vi "AddRecordingOverlay2Image.vi"(8 "error in (no error)":errorcluster, 10 "Recording Status String":string, 11 "Input Image":T1) -> (0 "error out":errorcluster, 3 "Output Image":T1)   [LabVIEW 2013]
doc: "Use this template to build a VI to use as a subVI."
uses:
  <vilib>/vision/Image Controls.llb/IMAQ Image.ctl
panel:
  out "Reference Image":T1(plugin-control)
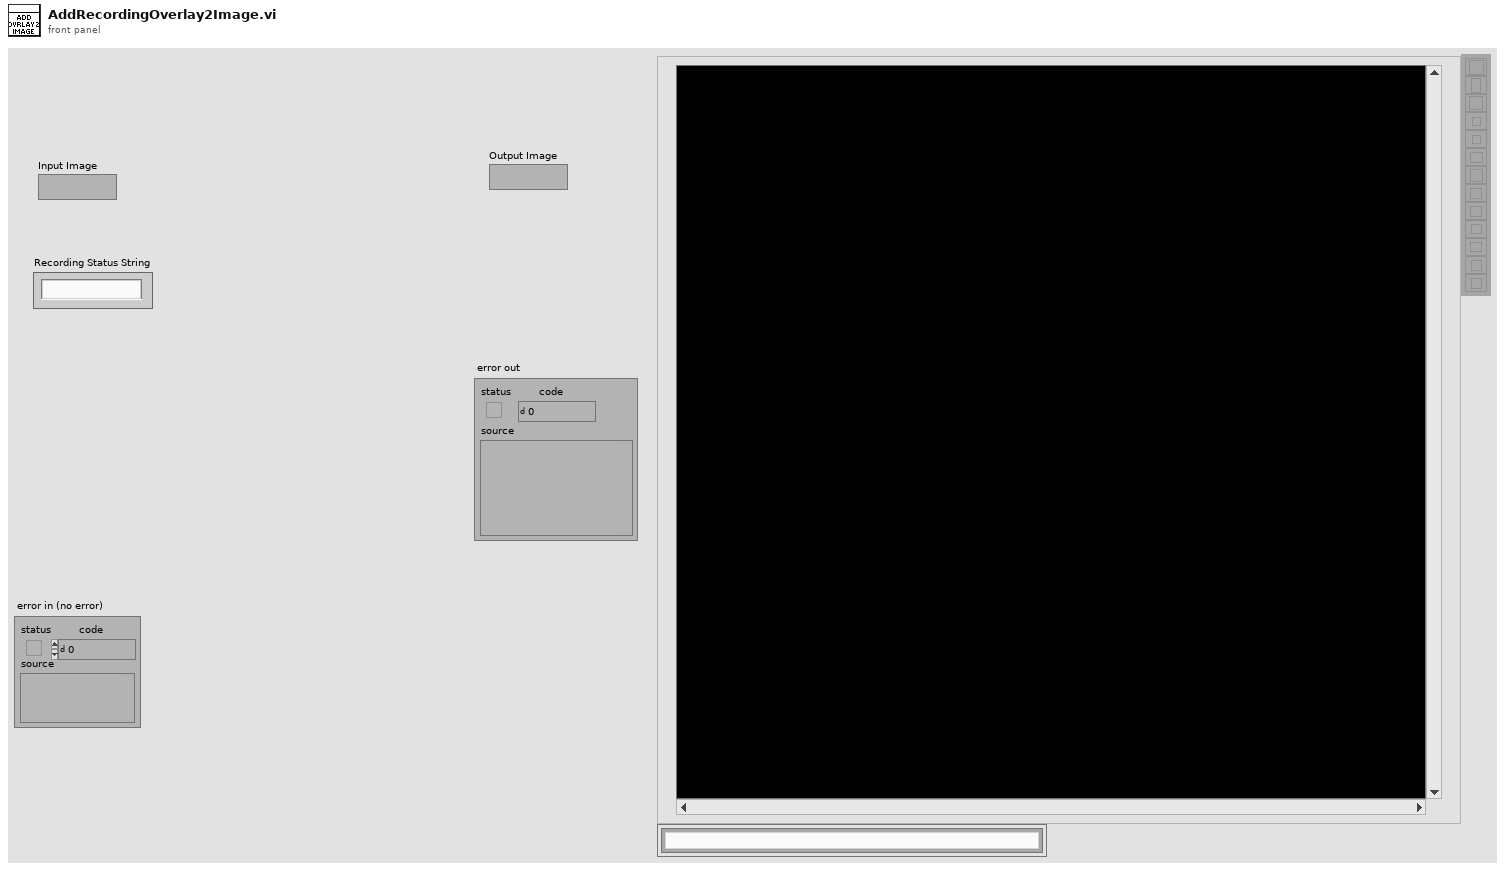
[diagram p1: front panel]
types:
  T1 = typedef "IMAQ Image.ctl" = refnum<image>
  T2 = cluster{"Left":i32, "Top":i32, "Right":i32, "Bottom":i32}
  T3 = cluster{"Desired Font (Application)":enum16{"User-specified Font", "Application Font", "System Font", "Dialog Font"}, "[User-specified Font]":cluster{"Font Name":string, "Size":i16, "Strikeout?":bool, "Italic?":bool, "Underline?":bool, "Outline?":bool, "Shadow?":bool, "Bold?":bool, "Rotation Angle":dbl}, "Horizontal Alignment":i16, "Vertical Alignment":i16}
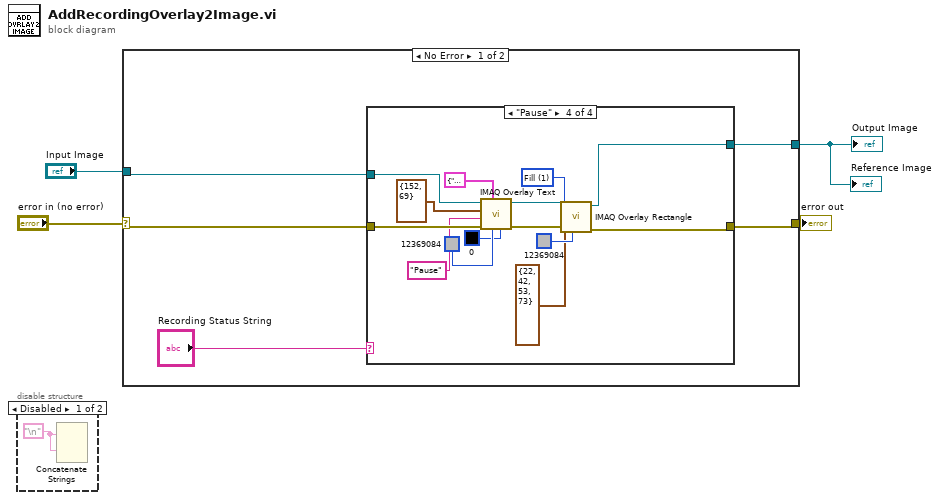
[diagram p0: block diagram]
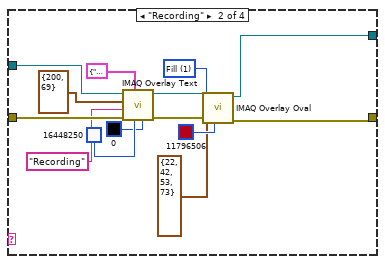
[diagram p4: hidden frame]
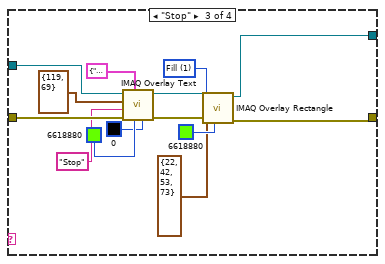
[diagram p5: hidden frame]
diagram:
  n1 = disable-structure shown="Disabled" {
    frame Disabled {
      w5 = "\n"
      n2 = Concatenate Strings(w5, w5) -> ()  [unwired: 3 in, 1 out]
    }
    frame Enabled {
    }
  }
  n3 = case shown="No Error" "error in (no error)" {
    selector: "error in (no error)" -> [w9 w55]
    tunnel: [w6 w55] -> w3
    tunnel: "Input Image" -> [w8 w54]
    tunnel: [w7 w54] -> w1
    frame No Error {
      n4 = case shown="\"Pause\"" "Recording Status String" {
        tunnel: w9 -> [_ w22 w36 w50]
        tunnel: w8 -> [w11 w21 w35 w49]
        tunnel: [w11 w15 w29 w43] -> w7
        tunnel: [_ w17 w31 w45] -> w6
        frame "False", Default {
        }
        frame "Recording" {
          w14 = u32 1 items=["Frame", "Fill"] ("Drawing Mode (Frame)")
          n5 = call "IMAQ Overlay Text"("BG Color (Transparent)"=u32 0, "Text Color (black)"=u32 16448250, "Font, Size & Style"=T3 {"Desired Font (Application)"=enum."User-specified Font", "[User-specified Font]"={"Font Name"="", "Size"=32, "Strikeout?"=FALSE, "Italic?"=FALSE, "Underline?"=FALSE, "Outline?"=FALSE, "Shadow?"=FALSE, "Bold?"=TRUE, "Rotation Angle"=0.0}, "Horizontal Alignment"=2, "Vertical Alignment"=2}, "error in (no error)"=w22, "String"="Recording", "Origin"=cluster{"X":i32, "Y":i32} {"X"=200, "Y"=69}, "Image"=w21) -> ("error out"=w18:errorcluster, "Image Out"=w16:T1)  [unwired: 3 in]
          n6 = call "IMAQ Overlay Oval"("Color"=u32 11796506, "error in (no error)"=w18, "Drawing Mode (Frame)"=w14, "Bounding Rectangle"=T2 {"Left"=22, "Top"=42, "Right"=53, "Bottom"=73}, "Image"=w16) -> ("error out"=w17:errorcluster, "Image Out"=w15:T1)  [unwired: 5 in]
        }
        frame "Stop" {
          w28 = u32 1 items=["Frame", "Fill"] ("Drawing Mode (Frame)")
          n7 = call "IMAQ Overlay Text"("BG Color (Transparent)"=u32 0, "Text Color (black)"=u32 6618880, "Font, Size & Style"=T3 {"Desired Font (Application)"=enum."User-specified Font", "[User-specified Font]"={"Font Name"="", "Size"=32, "Strikeout?"=FALSE, "Italic?"=FALSE, "Underline?"=FALSE, "Outline?"=FALSE, "Shadow?"=FALSE, "Bold?"=TRUE, "Rotation Angle"=0.0}, "Horizontal Alignment"=2, "Vertical Alignment"=2}, "error in (no error)"=w36, "String"="Stop", "Origin"=cluster{"X":i32, "Y":i32} {"X"=119, "Y"=69}, "Image"=w35) -> ("error out"=w32:errorcluster, "Image Out"=w30:T1)  [unwired: 3 in]
          n8 = call "IMAQ Overlay Rectangle"("Color"=u32 6618880, "error in (no error)"=w32, "Drawing Mode (Frame)"=w28, "Rectangle"=T2 {"Left"=22, "Top"=42, "Right"=53, "Bottom"=73} ("Bounding Rectangle"), "Image"=w30) -> ("error out"=w31:errorcluster, "Image Out"=w29:T1)  [unwired: 5 in]
        }
        frame "Pause" {
          w42 = u32 1 items=["Frame", "Fill"] ("Drawing Mode (Frame)")
          n9 = call "IMAQ Overlay Text"("BG Color (Transparent)"=u32 0, "Text Color (black)"=u32 12369084, "Font, Size & Style"=T3 {"Desired Font (Application)"=enum."User-specified Font", "[User-specified Font]"={"Font Name"="", "Size"=32, "Strikeout?"=FALSE, "Italic?"=FALSE, "Underline?"=FALSE, "Outline?"=FALSE, "Shadow?"=FALSE, "Bold?"=TRUE, "Rotation Angle"=0.0}, "Horizontal Alignment"=2, "Vertical Alignment"=2}, "error in (no error)"=w50, "String"="Pause", "Origin"=cluster{"X":i32, "Y":i32} {"X"=152, "Y"=69}, "Image"=w49) -> ("error out"=w46:errorcluster, "Image Out"=w44:T1)  [unwired: 3 in]
          n10 = call "IMAQ Overlay Rectangle"("Color"=u32 12369084, "error in (no error)"=w46, "Drawing Mode (Frame)"=w42, "Rectangle"=T2 {"Left"=22, "Top"=42, "Right"=53, "Bottom"=73} ("Bounding Rectangle"), "Image"=w44) -> ("error out"=w45:errorcluster, "Image Out"=w43:T1)  [unwired: 5 in]
        }
      }
    }
    frame Error {
    }
  }
  "error out" <- w3
  "Reference Image" <- w1
  "Output Image" <- w1
